vi "Scan Engine EtherCAT Slave.vi"(8 "error in (no error)":errorcluster, 11 "Node Ptr":T1 format="%.0x") -> (0 "error out":errorcluster)   [LabVIEW 2017, in "Scan Engine Custom Device.lvlib"]
uses:
  Scan Engine Custom Device.lvlib
  <vilib>/NI Veristand/Custom Device API/Custom Device Item Ref.ctl
  <vilib>/NI Veristand/Custom Device API/Custom Device API.lvlib
panel:
  in  "Prepend":bool caption="Prepend slave position to name"
  in  "SHDocVw.IWebBrowser2":refnum<k7>(container)
  in  "Slave Position":u16
  in  "Header":cluster{"Section Name":string}={"Section Name"="NI-9144 Chassis"}
  in  "Name":string
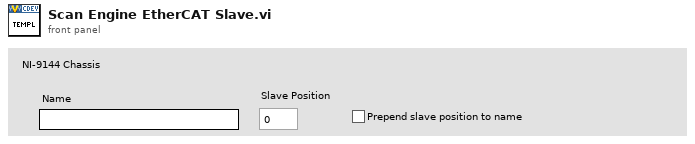
[diagram p1: front panel]
types:
  T1 = typedef "Custom Device API.lvlib/Custom Device Item Ref.ctl" = u64
  T2 = typedef "Custom Device API.lvlib/Custom Device Commands.ctl" = enum16{"Default", "Item renamed", "Shutdown", "Dynamic button pressed"}
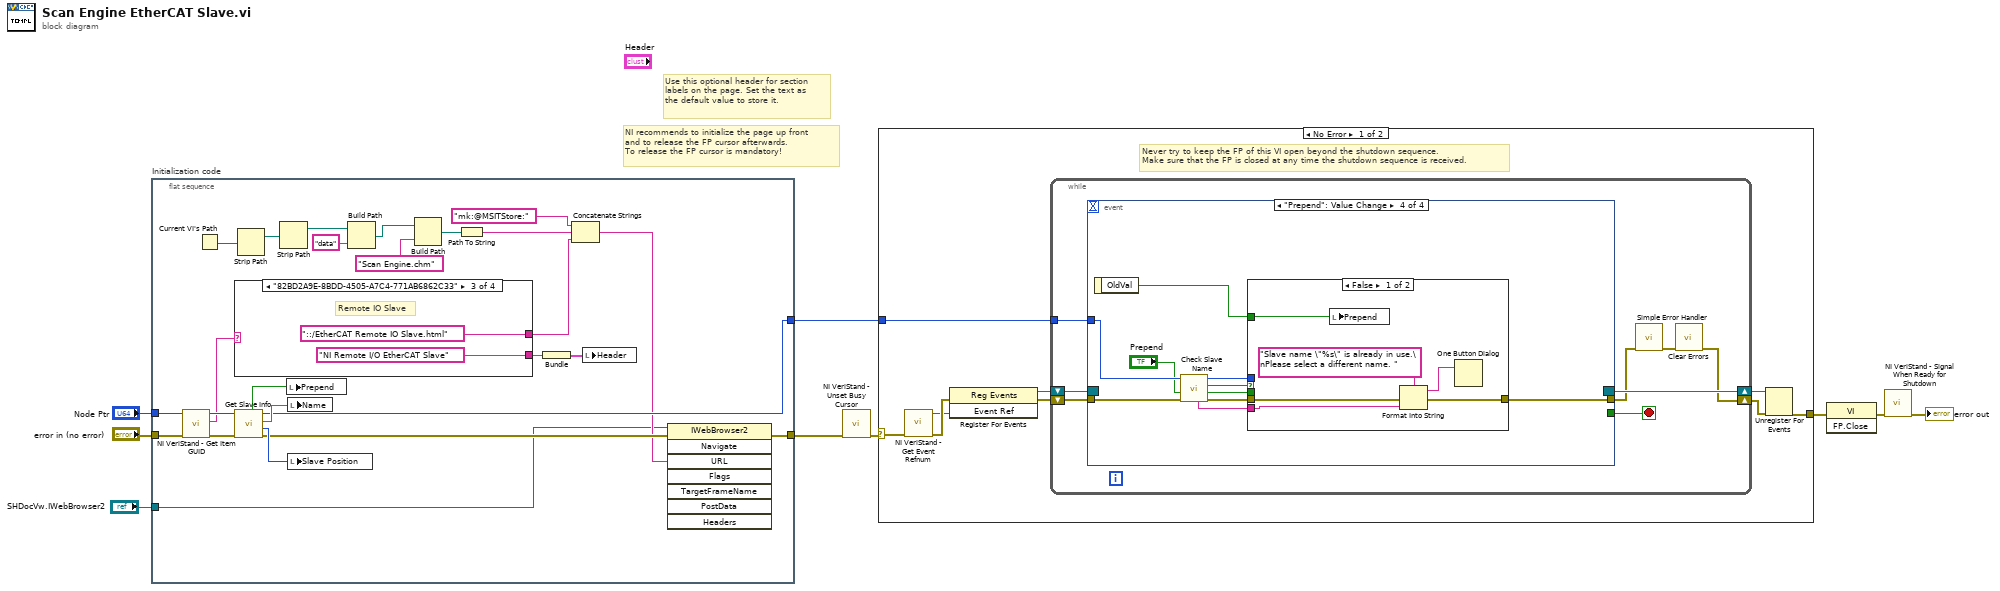
[diagram p0: block diagram]
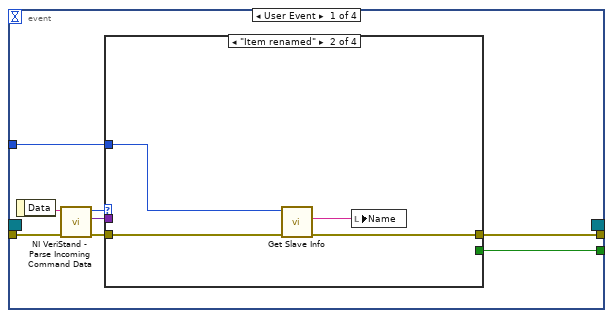
[diagram p2: hidden frame]
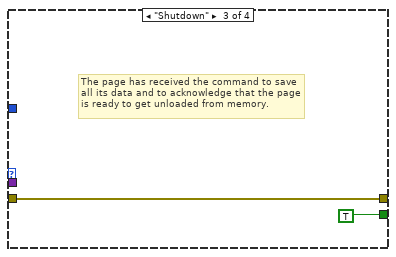
[diagram p4: hidden frame]
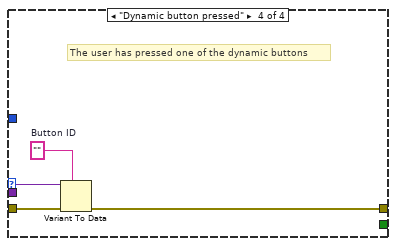
[diagram p5: hidden frame]
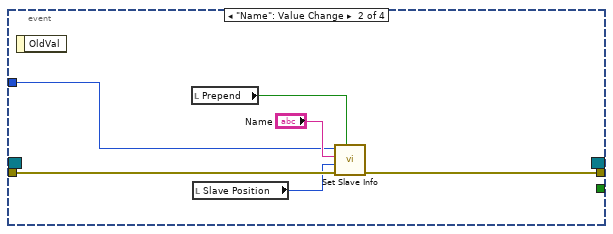
[diagram p6: hidden frame]
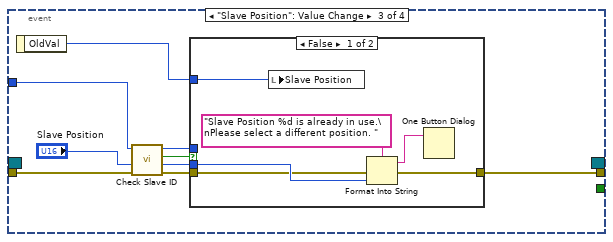
[diagram p7: hidden frame]
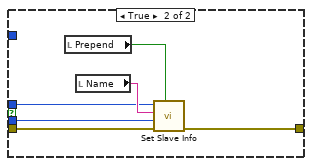
[diagram p8: hidden frame]
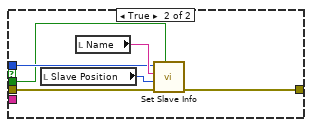
[diagram p9: hidden frame]
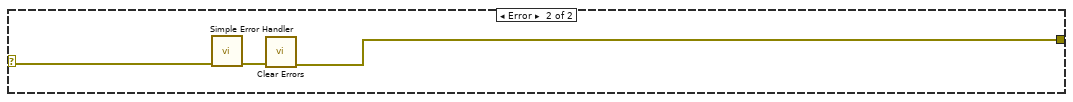
[diagram p10: hidden frame]
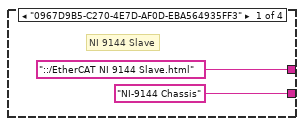
[diagram p11: hidden frame]
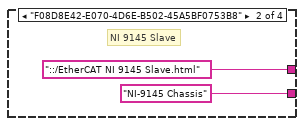
[diagram p12: hidden frame]
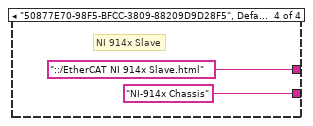
[diagram p13: hidden frame]
diagram:
  # "Use this optional header for section labels on the page. Set the text as the default value to store it."
  # "NI recommends to initialize the page up front\nand to release the FP cursor afterwards.\nTo release the FP cursor is mandatory!"
  n1 = flat-sequence "Initialization code" {
    tunnel: "error in (no error)" -> [w31]
    tunnel: "Node Ptr" -> [w15]
    tunnel: [w20] -> w5
    tunnel: [w32] -> w2
    tunnel: "SHDocVw.IWebBrowser2" -> [w18]
    frame #0 {
      n2 = call <vilib>:"NI VeriStand - Get Item GUID.vi"("error in (no error)"=w31, "Item Ref in"=w15) -> ("error out"=w16:errorcluster, "GUID"=w13:string, "Item Ref out"=w14:T1)  [unwired: 7 in]
      n3 = Current VI's Path() -> (path=w22:path)
      n4 = case shown="\"82BD2A9E-8BDD-4505-A7C4-771AB6862C33\"" w13 {
        tunnel: ["::/EtherCAT NI 9144 Slave.html" ("name or relative path") "::/EtherCAT NI 9145 Slave.html" ("name or relative path") "::/EtherCAT Remote IO Slave.html" ("name or relative path") "::/EtherCAT NI 914x Slave.html" ("name or relative path")] -> w12
        tunnel: ["NI-9144 Chassis" ("Section Name") "NI-9145 Chassis" ("Section Name") "NI Remote I/O EtherCAT Slave" ("Section Name") "NI-914x Chassis" ("Section Name")] -> w11
        frame "0967D9B5-C270-4E7D-AF0D-EBA564935FF3" {
          # "NI 9144 Slave"
        }
        frame "F08D8E42-E070-4D6E-B502-45A5BF0753B8" {
          # "NI 9145 Slave"
        }
        frame "82BD2A9E-8BDD-4505-A7C4-771AB6862C33" {
          # "Remote IO Slave"
        }
        frame "50877E70-98F5-BFCC-3809-88209D9D28F5", Default {
          # "NI 914x Slave"
        }
      }
      n5 = call "Get Slave Info.vi"("error in (no error)"=w16, "Item Ref in"=w14) -> ("error out"=w21:errorcluster, "Slave #"=w33:u16, "Slave Name"=w34:string, "Item Ref out"=w32:T1, "Prepend"=w17:bool)  [unwired: 5 in]
      n6 = Strip Path(path=w22) -> (stripped path=w23:path)  [unwired: 1 out]
      n7 = Strip Path(path=w23) -> (stripped path=w28:path)  [unwired: 1 out]
      n8 = local write "Prepend"(w17) -> ()
      n9 = local write "Name"(w34) -> ()
      n10 = local write "Slave Position"(w33) -> ()
      n11 = Build Path(base path=w28, name or relative path="data") -> (appended path=w29:path)
      n12 = Build Path(base path=w29, name or relative path="Scan Engine.chm") -> (appended path=w26:path)
      n13 = Path To String(path=w26) -> (string=w25:string)
      n14 = Bundle("Section Name"=w11) -> (w10:cluster{"Section Name":string})  [unwired: 1 in]
      n15 = Concatenate Strings("mk:@MSITStore:" ("string"), w25, w12) -> (w19:string)
      n16 = local write "Header"(w10) -> ()
      n17 = invoke class="IWebBrowser2" method="Navigate"(reference=w18, error in=w21, "URL"=w19) -> (error out=w20:errorcluster)  [unwired: 5 in, 7 out]
    }
  }
  n18 = call <vilib>:"NI VeriStand - Unset Busy Cursor.vi"("error in (no error)"=w5) -> ("error out"=w4:errorcluster)  [unwired: 10 out]
  n19 = case shown="No Error" w4 {
    selector: w4 -> [w43 w130]
    tunnel: [w48 w128] -> w9
    tunnel: w2 -> [w44 _]
    frame No Error {
      # "Never try to keep the FP of this VI open beyond the shutdown sequence.\nMake sure that the FP is closed at any time the shutdown sequence is received."
      n20 = call <vilib>:"NI VeriStand - Get Event Refnum.vi"("error in (no error)"=w43) -> ("error out"=w51:errorcluster, "Event Ref"=w47:refnum<user-event>)  [unwired: 9 out]
      n21 = register-events(error in=w51, w47) -> (reference out=w45:refnum<event-registration>, error out=w46:errorcluster)  [unwired: 1 in]
      n22 = while {
        tunnel: w44 -> [w55]
        shift-right: [w52] -> w49
        shift-left: w46 -> [w58]
        shift-right: [w59] -> w50
        shift-left: w45 -> [w57]
        stop <- w56 stop-if-true
        n23 = event shown="[3] \"Prepend\": Value Change" {
          selector: w57 -> [_ _ _ _]
          dyn-events: [_ _ _ _] -> w59
          timeout: _ -> [_ _ _ _]
          tunnel: w58 -> [w67 w82 w87 w113]
          tunnel: [w63 _ _ _] -> w56
          tunnel: [w62 w83 w85 w114] -> w54
          tunnel: w55 -> [w61 w81 w89 w112]
          event User Event {
            n24 = event-data() -> ("Data"=w66:string)  [unwired: 1 out]
            n25 = call <vilib>:"NI VeriStand - Parse Incoming Command Data.vi"("error in (no error)"=w67, "Incoming data"=w66) -> ("error out"=w65:errorcluster, "Outgoing data"=w60:variant, "Action"=w64:T2)  [unwired: 7 out]
            n26 = case shown="\"Item renamed\"" w64 {
              tunnel: w65 -> [w68 w72 w73 w78]
              tunnel: [_ _ TRUE _] -> w63
              tunnel: [w68 w71 w73 w75] -> w62
              tunnel: w61 -> [_ w69 _ _]
              tunnel: w60 -> [_ _ _ w77]
              frame "Default", Default {
              }
              frame "Item renamed" {
                n27 = call "Get Slave Info.vi"("error in (no error)"=w72, "Item Ref in"=w69) -> ("error out"=w71:errorcluster, "Slave Name"=w70:string)  [unwired: 5 in, 3 out]
                n28 = local write "Name"(w70) -> ()
              }
              frame "Shutdown" {
                # "The page has received the command to save all its data and to acknowledge that the page is ready to get unloaded from memory."
              }
              frame "Dynamic button pressed" {
                w76 = ""  # Button ID
                # "The user has pressed one of the dynamic buttons"
                n29 = Variant To Data(error in=w78, type=w76, Variant=w77) -> (error out=w75:errorcluster)  [unwired: 1 out]
              }
            }
          }
          event "Name": Value Change {
            n30 = event-data() -> ()  [unwired: 2 out]
            n31 = local read "Prepend"() -> (w79:bool)
            n32 = local read "Slave Position"() -> (w80:u16)
            n33 = call "Set Slave Info.vi"("Prepend"=w79, "error in (no error)"=w82, "Slave #"=w80, "Slave Name"="Name", "Item Ref in"=w81) -> ("error out"=w83:errorcluster)  [unwired: 5 in, 1 out]
          }
          event "Slave Position": Value Change {
            n34 = event-data() -> ("OldVal"=w86:u16)  [unwired: 1 out]
            n35 = call "Check Slave ID.vi"("error in (no error)"=w87, "Slave ID in"="Slave Position", "Item Ref in"=w89) -> ("error out"=w93:errorcluster, "Slave ID out"=w91:u16, "Available?"=w92:bool, "Item Ref out"=w90:T1)  [unwired: 5 in]
            n36 = case shown="False" w92 {
              tunnel: [w95 w105] -> w85
              tunnel: w93 -> [w96 w104]
              tunnel: w90 -> [_ w101]
              tunnel: w91 -> [w98 w103]
              tunnel: w86 -> [w94 _]
              frame False {
                n37 = local write "Slave Position"(w94) -> ()
                n38 = Format Into String(format string="Slave Position %d is already in use.\nPlease select a different position. ", error in=w96, w98) -> (resulting string=w97:string, error out=w95:errorcluster)  [unwired: 1 in]
                n39 = One Button Dialog(message=w97) -> ()  [unwired: 1 in, 1 out]
              }
              frame True {
                n40 = local read "Prepend"() -> (w100:bool)
                n41 = local read "Name"() -> (w102:string)
                n42 = call "Set Slave Info.vi"("Prepend"=w100, "error in (no error)"=w104, "Slave #"=w103, "Slave Name"=w102, "Item Ref in"=w101) -> ("error out"=w105:errorcluster)  [unwired: 5 in, 1 out]
              }
            }
          }
          event "Prepend": Value Change {
            n43 = event-data() -> ("OldVal"=w115:bool)  [unwired: 1 out]
            n44 = call "Check Slave Name.vi"("error in (no error)"=w113, "Prepend in"="Prepend", "Item Ref in"=w112) -> ("error out"=w108:errorcluster, "Prepend out"=w107:bool, "Available?"=w109:bool, "Item Ref out"=w110:T1, "Slave Name"=w106:string)  [unwired: 4 in]
            n45 = case shown="False" w109 {
              tunnel: [w118 w127] -> w114
              tunnel: w108 -> [w119 w126]
              tunnel: w110 -> [_ w124]
              tunnel: w107 -> [_ w123]
              tunnel: w115 -> [w121 _]
              tunnel: w106 -> [w116 _]
              frame False {
                n46 = local write "Prepend"(w121) -> ()
                n47 = Format Into String(format string="Slave name \"%s\" is already in use.\nPlease select a different name. ", error in=w119, w116) -> (resulting string=w117:string, error out=w118:errorcluster)  [unwired: 1 in]
                n48 = One Button Dialog(message=w117) -> ()  [unwired: 1 in, 1 out]
              }
              frame True {
                n49 = local read "Slave Position"() -> (w122:u16)
                n50 = local read "Name"() -> (w125:string)
                n51 = call "Set Slave Info.vi"("Prepend"=w123, "error in (no error)"=w126, "Slave #"=w122, "Slave Name"=w125, "Item Ref in"=w124) -> ("error out"=w127:errorcluster)  [unwired: 5 in, 1 out]
              }
            }
          }
        }
        n52 = call <vilib>:"Simple Error Handler.vi"("error in (no error)"=w54) -> ("error out"=w53:errorcluster)  [unwired: 1 in, 7 out]
        n53 = call <vilib>:"Clear Errors.vi"("error in (no error)"=w53) -> ("error out"=w52:errorcluster)  [unwired: 1 in, 5 out]
      }
      n54 = Unregister For Events(event registration refnum=w50, error in=w49) -> (error out=w48:errorcluster)
    }
    frame Error {
      n55 = call <vilib>:"Simple Error Handler.vi"("error in (no error)"=w130) -> ("error out"=w129:errorcluster)  [unwired: 1 in, 7 out]
      n56 = call <vilib>:"Clear Errors.vi"("error in (no error)"=w129) -> ("error out"=w128:errorcluster)  [unwired: 1 in, 5 out]
    }
  }
  n57 = invoke class="VI" method="FP.Close"(error in=w9) -> (error out=w8:errorcluster)  [unwired: 2 in, 2 out]
  n58 = call <vilib>:"NI VeriStand - Signal When Ready for Shutdown.vi"("error in (no error)"=w8) -> ("error out"=→"error out":errorcluster)  [unwired: 10 out]
